vi "cblas dgemm.vi"(0 "A":T3, 1 "B":T3, 2 "C":T3, 3 "alpha":dbl=1.0, 4 "beta":dbl=1.0, 5 "order":T1=101 items=["CblasRowMajor"=101, "CblasColMajor"=102], 6 "transA":T2=111 items=["CblasNoTrans"=111, "CblasTrans"=112, "CblasConjTrans "=113], 7 "transB":T2=111 items=["CblasNoTrans"=111, "CblasTrans"=112, "CblasConjTrans "=113], 8 "lda":i32, 9 "m":i32=-1, 10 "ldb":i32, 11 "n":i32=-1, 12 "ldc":i32, 13 "k":i32=-1) -> (14 "dgemm":T3, 19 "error":i32)   [LabVIEW 2017, in "NI_AALBLAS.lvlib"]
uses:
  NI_AALBLAS.lvlib
  RealMatrix.ctl
  Operation_Transpose.ctl
  Order.ctl
  NI_Matrix.lvlib
  lvblas.dll
panel:
  # "void cblas_dgemm(order, transA, transB, m, n, k, alpha,*A, lda, *B, ldb, beta, *C, ldc)"
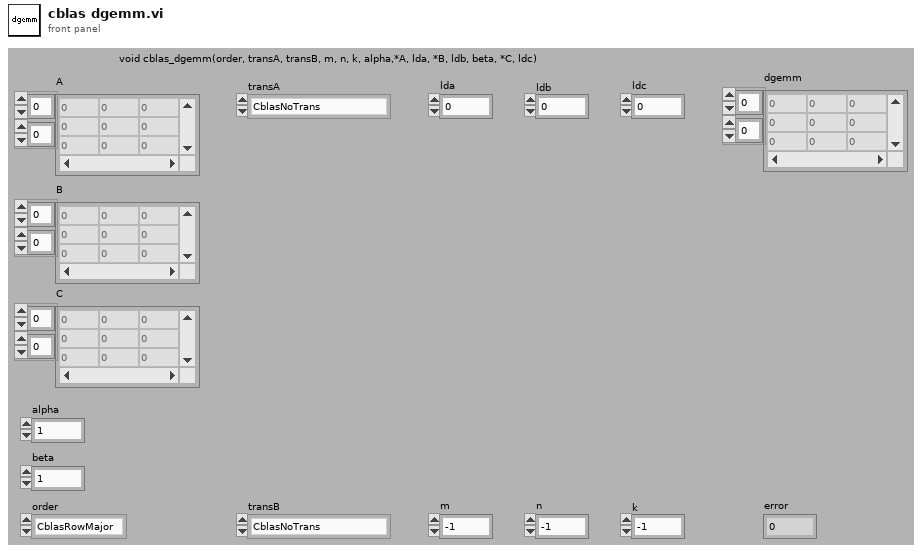
[diagram p1: front panel]
types:
  T1 = typedef "NI_AALBLAS.lvlib/Order.ctl" = i32
  T2 = typedef "NI_AALBLAS.lvlib/Operation_Transpose.ctl" = i32
  T3 = typedef "NI_Matrix.lvlib/RealMatrix.ctl" = dbl[][]
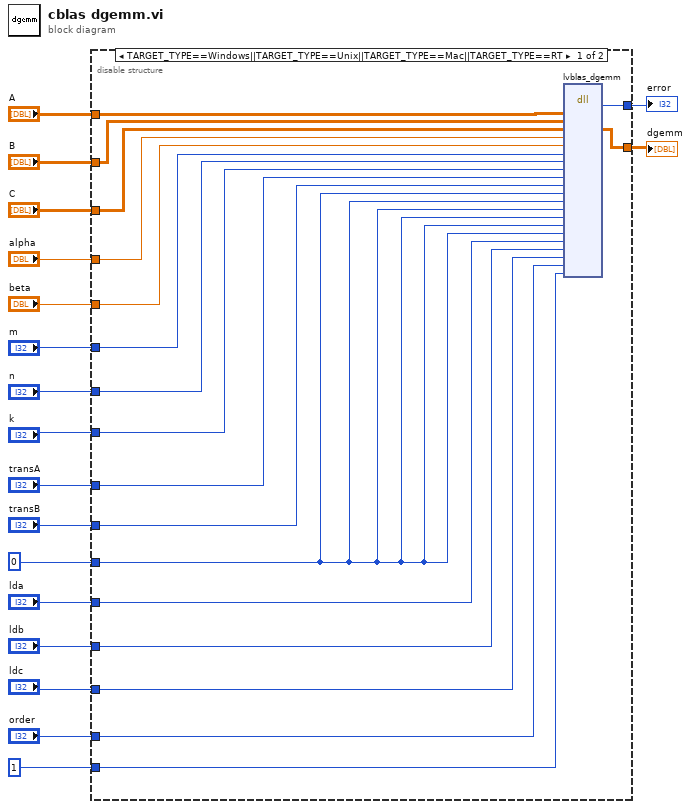
[diagram p0: block diagram]
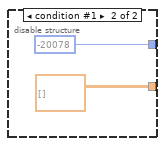
[diagram p2: hidden frame]
diagram:
  n1 = disable-structure shown="TARGET_TYPE==Windows||TARGET_TYPE==Unix||TARGET_TYPE==Mac||TARGET_TYPE==RT" {
    disable-tunnel: [w36 -20078 ("error")] -> w18
    disable-tunnel: "A" -> [w35 _]
    disable-tunnel: "B" -> [w34 _]
    disable-tunnel: "C" -> [w33 _]
    disable-tunnel: "alpha" -> [w32 _]
    disable-tunnel: "beta" -> [w31 _]
    disable-tunnel: [w30 T3 [] ("C")] -> w12
    disable-tunnel: "transB" -> [w29 _]
    disable-tunnel: 0 -> [w28 _]
    disable-tunnel: "transA" -> [w27 _]
    disable-tunnel: "order" -> [w26 _]
    disable-tunnel: "m" -> [w25 _]
    disable-tunnel: "n" -> [w24 _]
    disable-tunnel: "k" -> [w23 _]
    disable-tunnel: "lda" -> [w22 _]
    disable-tunnel: "ldb" -> [w21 _]
    disable-tunnel: "ldc" -> [w20 _]
    disable-tunnel: 1 -> [w19 _]
    frame condition #0 (active) {
      n2 = dll-call lib="C:/Program Files/National Instruments/LabVIEW 2017/resource/lvblas.*" fn="lvblas_dgemm" ("CBLAS.dll:MtrxxMtrxH")("A"=w35, "B"=w34, "C"=w33, "alpha"=w32, "beta"=w31, "m"=w25, "n"=w24, "k"=w23, "OpA"=w27, "OpB"=w29, "startARow"=w28, "startACol"=w28, "startBRow"=w28, "startBCol"=w28, "startCRow"=w28, "startCCol"=w28, "lda"=w22, "ldb"=w21, "ldc"=w20, "order"=w26, "check"=w19) -> ("error"=w36:i32, "C"=w30:dbl[][])  [unwired: 23 in, 2 out]
    }
    frame condition #1 {
    }
  }
  "dgemm" <- w12
  "error" <- w18
